vi "speed_radail0611.vi"(6 "XYZ Data":cluster{"X":dbl[], "Y":dbl[], "Z":dbl[]}, 7 "rate":dbl=10000.0, 8 "Optical":dbl, 9 "Pole Pair":i32=24, 10 "Voltage":dbl[](array[numeric])) -> (1 "B-EMF":dbl[](graph)=[0.07481589133166745, 0.07511337105786742, 0.0741529055838003, 0.07537265906376046, 0.07508825632115766, 0.07557435638030187, 0.0743975577603694, 0.07492228255252237, 0.07463056189525759, 0.0758438201846894, 0.07482290613743812, 0.07511679185821236, 0.07415273237871953, 0.07537876454285714, 0.07509791250440986, 0.07558596112071256, 0.0743927080181082, 0.07491881845090724, 0.07463770660483883, 0.07585304335523971, 0.07481316335164553, 0.07513961162760209, 0.07414004510655407, 0.0753934869747215, 0.07509271635198714, 0.07559592041285612, 0.07439296782572931, 0.07493276145990817, 0.07463588795149087, 0.07587720546400528, 0.07480203492520691, 0.07514974412482635, 0.07413324680713437, 0.07542358135750299, 0.07508440250811083, 0.07560570649991886, 0.07438603962249907, 0.07495536472294693, 0.07461891385357669, 0.07588144898848384, 0.07480381027728465, 0.07516195508301972, 0.07413138485251623, 0.07541942443556485, 0.07507565565153261, 0.07562294040545418, 0.07437421837573739, 0.07496484770111837, 0.07462229135265147, 0.07589993863085463, 0.07480216482901747, 0.07518568417908342, 0.07412164206672368, 0.07543691814872129, 0.07506110642474902, 0.07564398482276614, 0.07437668654813819, 0.07498160529268162, 0.07461267847066942, 0.0759097247179174, 0.07477362929196277, 0.07519404132422994, 0.07411445405587225, 0.07546108025748688, 0.07506634587844192, 0.07565281828188475, 0.07436131459722098, 0.07499658753216708, 0.07460471103695462, 0.07593150525682257, 0.0747739324008541, 0.07521118862722488, 0.07411661911938174, 0.075469350800093, 0.07505032440847191, 0.07567741340335221, 0.07435451629780128, 0.07502092284601342, 0.07459782613499454, 0.0759478731369541, 0.07476483913411439, 0.07523058759626963, 0.07409336633729012, 0.07548000291255955, 0.07504733662082885, 0.07569139971362333, 0.07435061918348428, 0.0750335235156385, 0.0745818912675649, 0.07596948047077853, 0.07476141833376944, 0.07525267124406612, 0.07408821348613759, 0.07550827864199311, 0.07503378332325962, 0.07571058217631717, 0.07433632976432183, 0.07505898466250974, 0.0745710659500176, 0.07598351008231984, 0.07475838724485617, 0.07526722047084973, 0.07407912021939786, 0.07552399700307182, 0.07501602980248206, 0.07573383495840878, 0.0743232094794545, 0.07508344988016666, 0.07455508778131775, 0.07600464110217219, 0.07473353231576757, 0.07529501988631122, 0.07406253583291537, 0.0755460806508683, 0.07500832217638835, 0.07575197819061805, 0.07430298778627613, 0.07510068378570196, 0.0745526629101872, 0.07604226990596659, 0.0747173376407168, 0.07531303321470993, 0.07405010836837107, 0.07557439968157206, 0.074991304777204, 0.07578306850261392, 0.07429489044875075, 0.0751250624008185, 0.07452858740396197, 0.07605456746670036, 0.07470581950284645, 0.0753423914758982, 0.07402646587484775, 0.07559358214426588, 0.07497147279545732, 0.07580671099613724, 0.07426800035996324, 0.07516173857666877, 0.07450693676886735, 0.07607426954463645, 0.07468577101474887, 0.07537097031422309, 0.07399957578606026, 0.07563593078651094, 0.07496328885539158, 0.0758321721430085, 0.07424877459599921, 0.07519157315182916, 0.07447896414832511, 0.07611419331575092, 0.07466234502757649, 0.07539301066074941, 0.07397181967186896, 0.07566411991340413, 0.07492154643092916, 0.07586607703756665, 0.0742194596360811, 0.07522162423334047, 0.07445055851508102, 0.07615680176561711, 0.07463056189525759, 0.07543172199629856, 0.07394415016021806, 0.07570560253024541, 0.0748928376887937, 0.07590998452553853, 0.07418278346023084, 0.07526743697720066, 0.07441184717953182, 0.07620157527899274, 0.07459211036732954, 0.0754861949941966, 0.07390513571577755, 0.075761114758628, 0.07485213449481584, 0.07596172954341465, 0.07414134414465974, 0.07530259760859431, 0.0], 2 "Speed(rad/s)":dbl[](graph), 3 "Acc Speed (rad/sec)":dbl[](array[numeric]), 4 "Voltage Data":dbl[](graph), 5 "output Data":T1)   [LabVIEW 2013]
uses:
  <vilib>/Math Plots/3D Math Plots/3D Scatter/3D Scatter XCtrl/3D Scatter.xctl
  <vilib>/Math Plots/3D Math Plots/3D Scatter/3D Scatter Datatype/Public/Plot Helper (Vector).vi
  <vilib>/gmath/interp.llb/Interpolate 2D Scattered (2D).vi
  <vilib>/Analysis/NI_AALBase.lvlib
  <vilib>/gmath/NI_AAL_Interpolation.lvlib
  <vilib>/Math Plots/3D Math Plots/3D Scatter/3D Scatter Datatype/3D Scatter Datatype.lvclass
panel:
  out "Raw Data 2":refnum<class "3D Plot Datatype.lvclass">[](xcontrol)
  out "min index(es)":i32
  out "Voltage Data 2":dbl[][](graph)
  out "Optical Torque":dbl
  out "speed":dbl format="%0.2f"
  in  "Cutoff Frequency":i32=1000
  out "Torque":dbl format="%.5f"
  out "Air gap distance":dbl
  in  "Data Change":bool=TRUE
  out "K Mean":dbl=0.07460512010090932
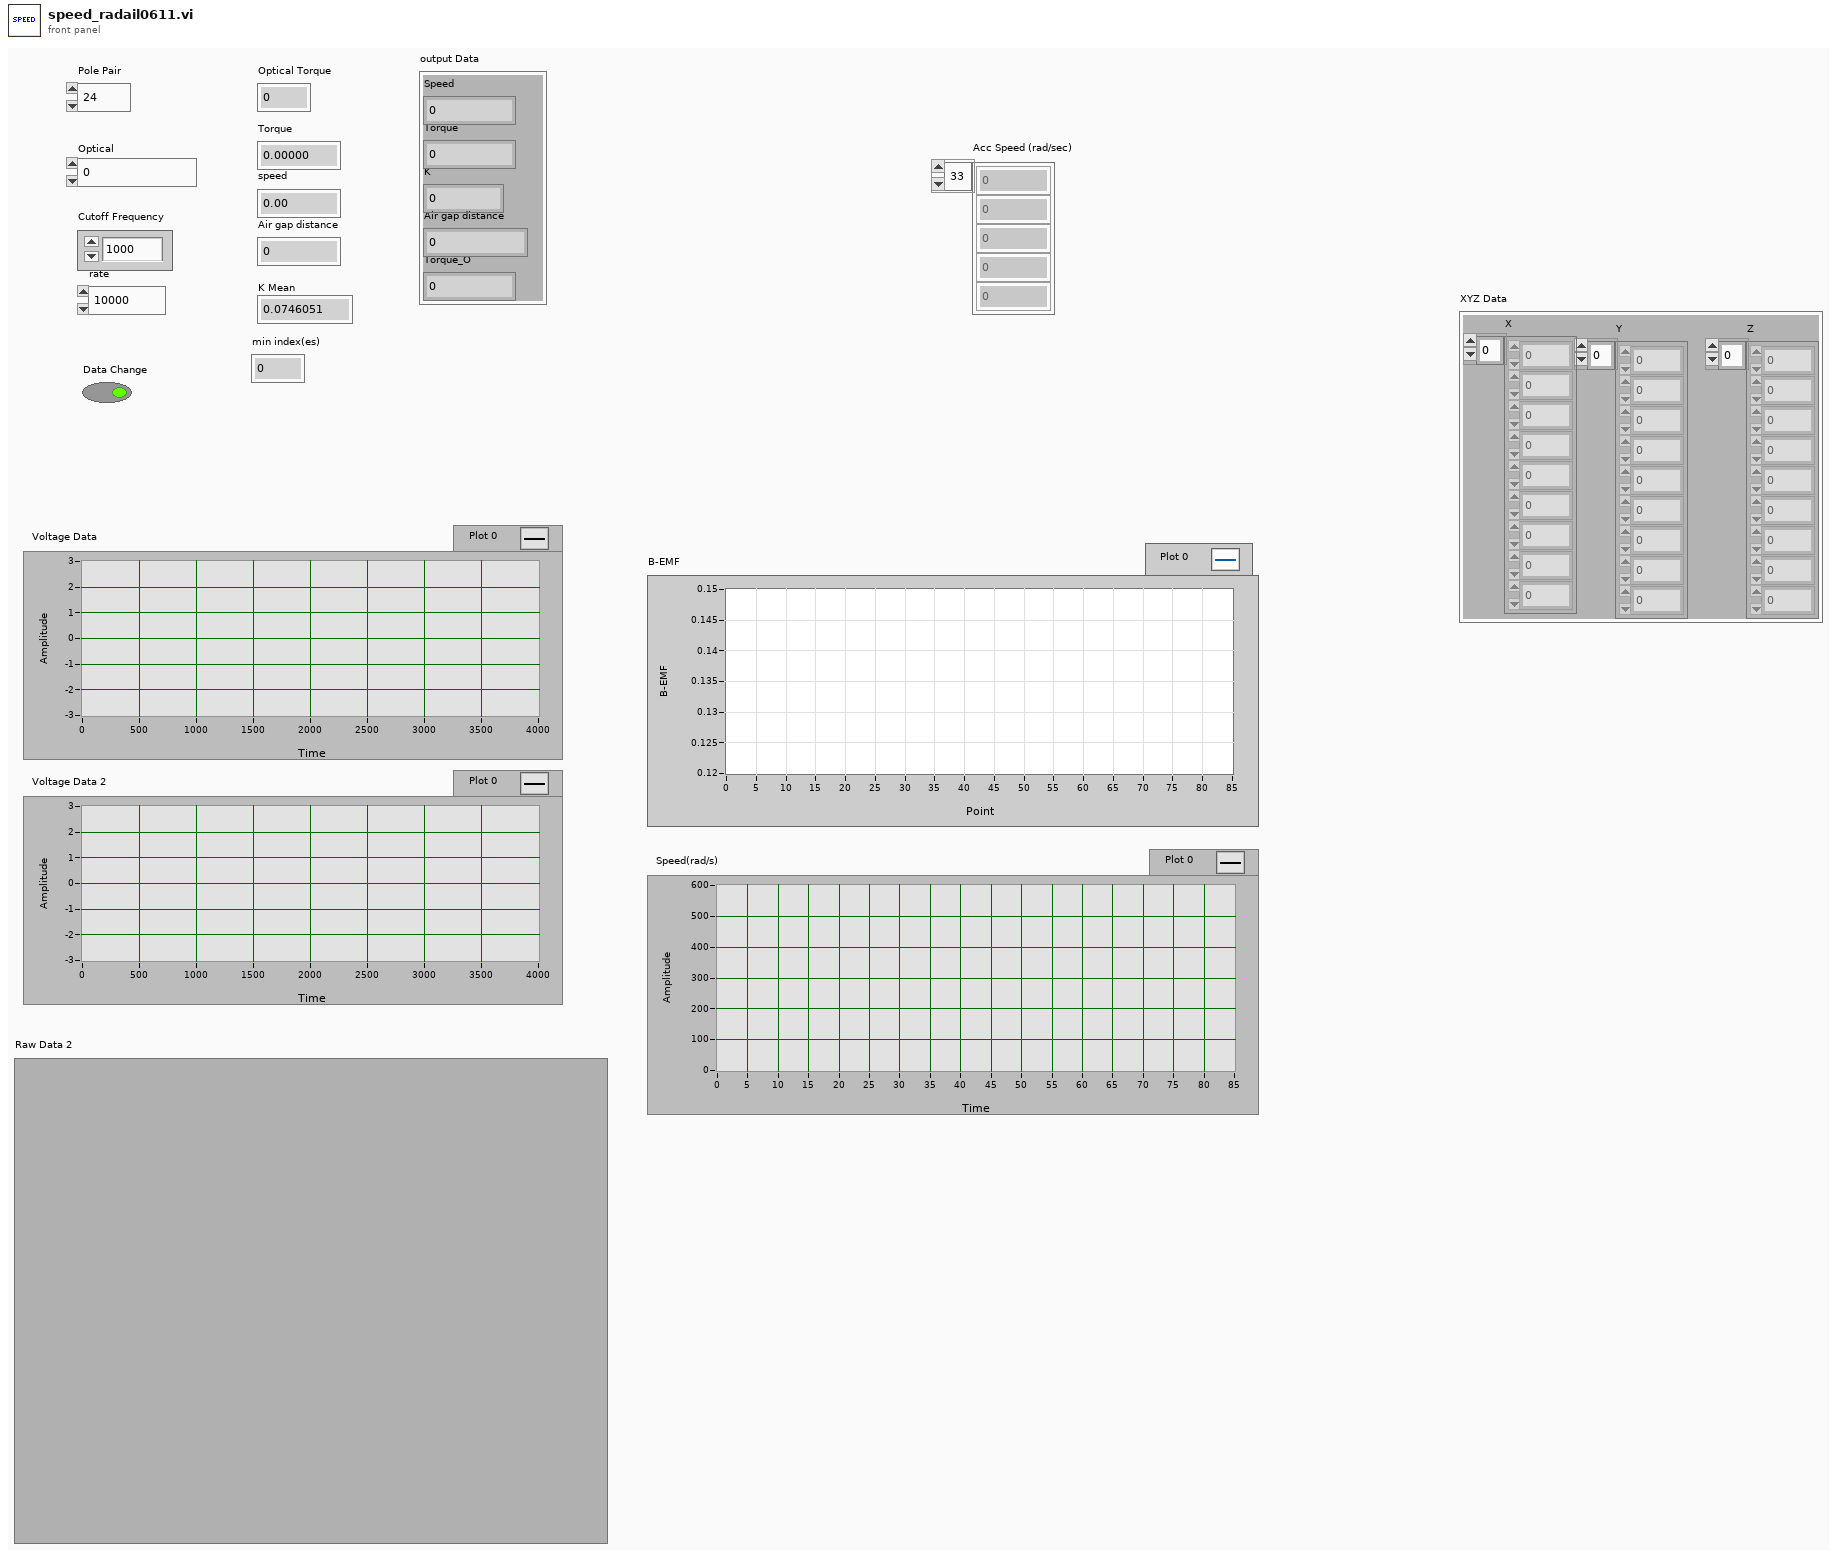
[diagram p1: front panel]
types:
  T1 = cluster{"Speed":dbl, "Torque":dbl, "K":dbl, "Air gap distance ":dbl, "Torque_O":dbl}
  T2 = cluster{"mean":dbl, dbl, "mean":dbl, "mean":dbl, dbl}
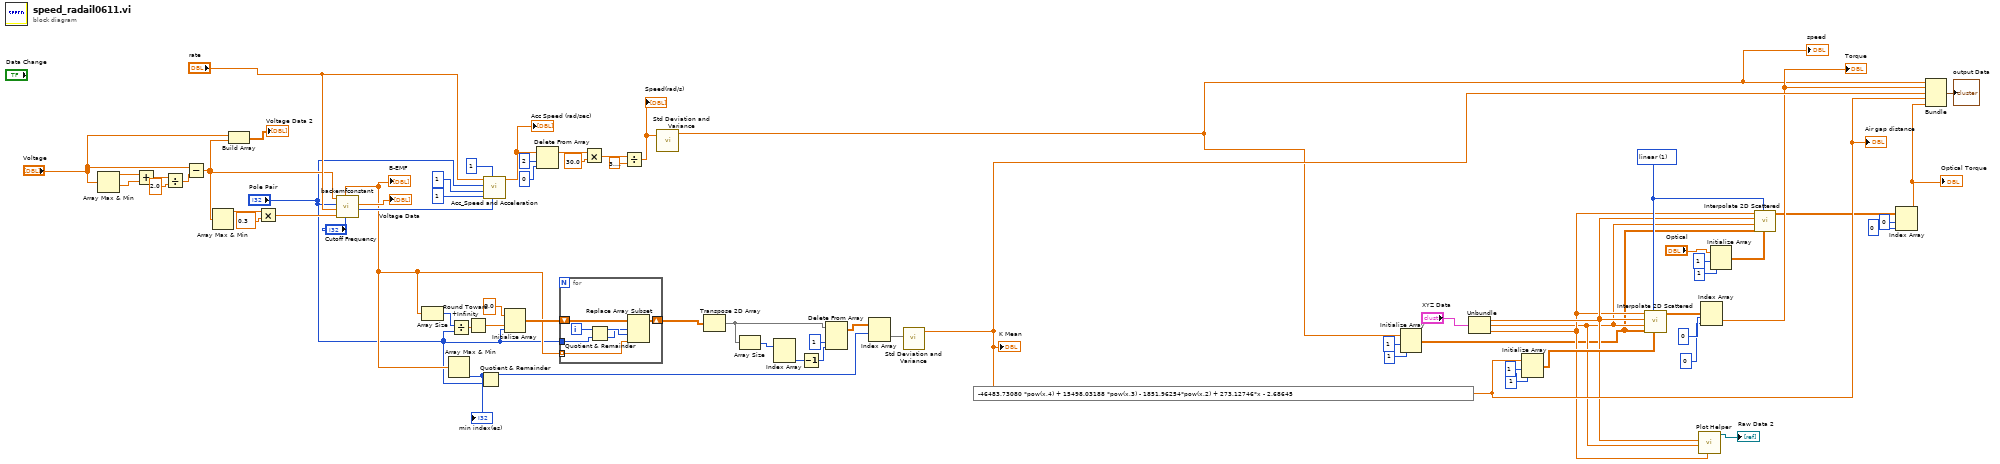
[diagram p0: block diagram]
diagram:
  w16 = 1 items=["nearest", "linear", "cubic", "biharmonic spline "] ("method")
  n1 = Array Max & Min(array="Voltage") -> (max value=w57:dbl, min value=w56:dbl)  [unwired: 2 out]
  n2 = Add(x=w57, y=w56) -> (x+y=w55:dbl)
  n3 = Divide(x=w55, y=2.0) -> (x/y=w46:dbl)
  n4 = Subtract(x="Voltage", y=w46) -> (x-y=w45:dbl[])
  n5 = Array Max & Min(array=w45) -> (max value=w51:dbl)  [unwired: 3 out]
  n6 = Build Array("Voltage", w45) -> (→"Voltage Data 2":dbl[][])
  n7 = Multiply(x=w51, y=0.3) -> (x*y=w67:dbl)
  n8 = call "backemfconstant.vi"("Cutoff Frequency"="Cutoff Frequency", "Noise Band"=w67, "rate"="rate", "Pole Pair"="Pole Pair", "Back  EMF data"=w45) -> ("ZCP"=w66:i32[], "Filiter Voltage"=→"Voltage Data":dbl[], "B-EMF"=w33:dbl[])  [unwired: 2 out]
  "B-EMF" <- w33
  n9 = Array Size(array=w33) -> (size(s)=w44:i32)
  n10 = Array Max & Min(array=w33) -> (min index (indices)=w32:i32)  [unwired: 3 out]
  "min index(es)" <- w32
  n11 = Divide(x=w44, y="Pole Pair") -> (x/y=w43:dbl)
  n12 = Round Toward +Infinity(x=w43) -> (ceil(x): smallest int >= x=w41:dbl)
  n13 = Quotient & Remainder(x=w32, y="Pole Pair") -> (x-y*floor(x/y)=w29:i32)  [unwired: 1 out]
  n14 = call "Acc_Speed and Acceleration.vi"("Count"=w66, "Encoder reduction"=1, "A_Gain"=1, "V_Gain"=1, "Pulse per rev."="Pole Pair", "Rate"="rate") -> ("Acc Speed (rad/sec)"=w65:dbl[])  [unwired: 3 out]
  "Acc Speed (rad/sec)" <- w65
  n15 = Initialize Array(0.0 ("element"), w41, "Pole Pair") -> (w40:dbl[][])
  n16 = Delete From Array(array=w65, length=2, index=0) -> (array with subset deleted=w59:dbl[])  [unwired: 1 out]
  n17 = for {
    tunnel: w33 -> [w72] mode=indexing
    shift-right: [w77] -> w39
    shift-left: w40 -> [w78]
    tunnel: "Pole Pair" -> [w75]
    i -> [w76]
    n18 = Quotient & Remainder(x=w76, y=w75) -> (x-y*floor(x/y)=w74:i32, floor(x/y)=w73:i32)
    n19 = Replace Array Subset(array=w78, new element=w72, index (row)=w73, index (col)=w74) -> (w77:dbl[][])
  }
  n20 = Multiply(x=w59, y=30.0) -> (x*y=w61:dbl[])
  n21 = Divide(x=w61, y=3.141592653589793) -> (x/y=w58:dbl[])
  "Speed(rad/s)" <- w58
  n22 = call <vilib>:"Std Deviation and Variance.vi"("X"=w58) -> ("mean"=w1:dbl)  [unwired: 1 in, 2 out]
  "speed" <- w1
  n23 = Transpose 2D Array(2D array=w39) -> (transposed array=w36:dbl[][])
  n24 = Array Size(array=w36) -> (size(s)=w38:i32[])
  n25 = Index Array(array=w38) -> (element #2=w37:i32)  [unwired: 2 in, 1 out]
  n26 = Decrement(x=w37) -> (x-1=w34:i32)
  n27 = Delete From Array(array=w36, length=1, index (col)=w34) -> (array with subset deleted=w31:dbl[][])  [unwired: 1 in, 1 out]
  n28 = Index Array(array=w31, index (row)=w29) -> (element=w30:dbl[])  [unwired: 1 in]
  n29 = call <vilib>:"Std Deviation and Variance.vi"("X"=w30) -> ("mean"=w24:dbl)  [unwired: 1 in, 2 out]
  "K Mean" <- w24
  n30 = expression code="-46483.73080 *pow(x,4) + 15498.03188 *pow(x,3) - 1851.96254*pow(x,2) + 273.12746*x - 2.68645"(w24) -> (w27:dbl)
  "Air gap distance" <- w27
  n31 = Initialize Array(w1, 1 ("dimension size"), 1 ("dimension size")) -> (w3:dbl[][])
  n32 = Unbundle("XYZ Data") -> ("X"=w6:dbl[], "Y"=w4:dbl[], "Z"=w5:dbl[])
  n33 = Initialize Array(w27, 1 ("dimension size"), 1 ("dimension size")) -> (w18:dbl[][])
  n34 = call-poly <vilib>:"Interpolate 2D Scattered.vi"("Yi"=w18, "method"=w16, "Xi"=w3, "Y"=w4, "X"=w6, "Z"=w5) -> ("Zi"=w21:dbl[][])  [unwired: 4 in, 1 out]
  n35 = call-poly <vilib>:"Plot Helper.vi"("z vector"=w5, "y vector"=w4, "x vector"=w6) -> ("3D Plot lvclass Array out"=→"Raw Data 2":refnum<class "3D Plot Datatype.lvclass">[])  [unwired: 3 in, 5 out]
  n36 = Index Array(array=w21, index (row)=0, index (col)=0 ("disabled index (col)")) -> (element=w17:dbl)
  "Torque" <- w17
  n37 = Initialize Array("Optical", 1 ("dimension size"), 1 ("dimension size")) -> (w12:dbl[][])
  n38 = call-poly <vilib>:"Interpolate 2D Scattered.vi"("Yi"=w12, "method"=w16, "Xi"=w3, "Y"=w4, "X"=w6, "Z"=w5) -> ("Zi"=w9:dbl[][])  [unwired: 4 in, 1 out]
  n39 = Index Array(array=w9, index (row)=0, index (col)=0 ("disabled index (col)")) -> (element=w8:dbl)
  "Optical Torque" <- w8
  n40 = Bundle("mean"=w1, w17, "mean"=w24, "mean"=w27, w8) -> (→"output Data":T2)  [unwired: 1 in]
